vi "DHE_SetControllerParams.vi"(9 "framesperbuffer":i32, 10 "ControllerStatus":T1={"Response"="", "power"=FALSE, "shutter"=FALSE, "artifdata"=FALSE, "idlemode"=FALSE, "reset"=FALSE, "gain"=0, "speed"=0, "resetPCI"=FALSE, "autoshutter"=FALSE, "TempSetPoint"=-110, "multipleextensions"=FALSE, "displayImage"=TRUE, "coadding"=FALSE, "images being coadded"=1, "Operation Mode"=enum."normal", "frames to write"={"subs"=FALSE, "reset"=FALSE, "exposed"=FALSE}, "fawler samples"=1, "write auto"=FALSE, "datatype"="", "frames to display"={"subs"=FALSE, "reset"=FALSE, "exposed"=FALSE}, "sur"=1, "autoclear"=FALSE}) -> ()   [LabVIEW 2016]
uses:
  Common/public/vis/CMN_ContStatus.ctl
  DBSHAND/private/vis/DatabaseHand_Element_Set(bool).vi
  DBSHAND/private/vis/DatabaseHand_Element_Set(U8).vi
  DBSHAND/private/vis/DatabaseHand_Element_Set(I32).vi
  DBSHAND/private/vis/DatabaseHand_Element_Set(string).vi
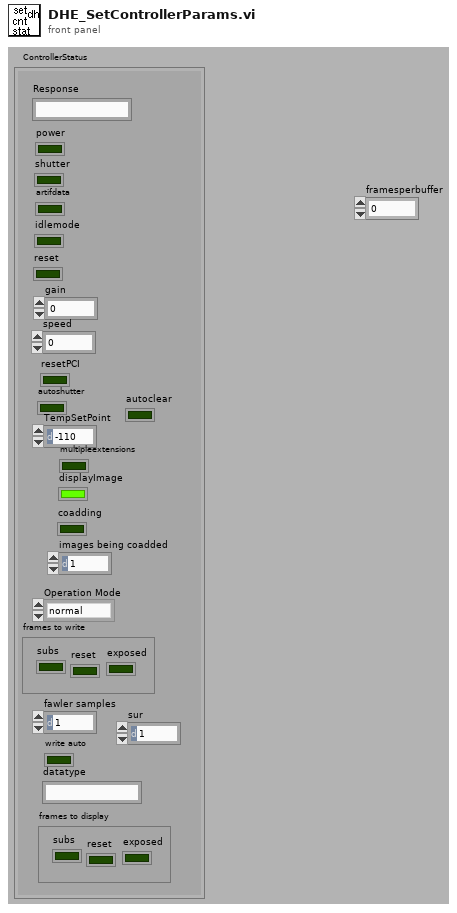
[diagram p1: front panel]
types:
  T1 = typedef "CMN_ContStatus.ctl" = cluster{"Response":string, "power":bool, "shutter":bool, "artifdata":bool, "idlemode":bool, "reset":bool, "gain":u8, "speed":u8, "resetPCI":bool, "autoshutter":bool, "TempSetPoint":i32, "multipleextensions":bool, "displayImage":bool, "coadding":bool, "images being coadded":i32, "Operation Mode":enum16{"normal", "coadd", "fawler"}, "frames to write":cluster{"subs":bool, "reset":bool, "exposed":bool}, "fawler samples":i32, "write auto":bool, "datatype":string, "frames to display":cluster{"subs":bool, "reset":bool, "exposed":bool}, "sur":i32, "autoclear":bool}
  T2 = typedef "DatabaseHand_RefNum.ctl" = refnum<vi>
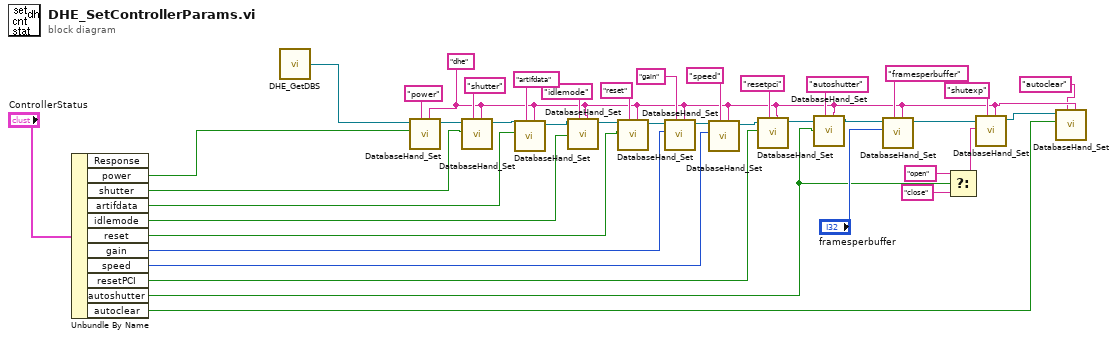
[diagram p0: block diagram]
diagram:
  w2 = "dhe" ("group")
  n1 = Unbundle By Name("ControllerStatus") -> ("power"=w38:bool, "shutter"=w32:bool, "artifdata"=w30:bool, "idlemode"=w28:bool, "reset"=w26:bool, "gain"=w16:u8, "speed"=w15:u8, "resetPCI"=w25:bool, "autoshutter"=w8:bool, "autoclear"=w3:bool)  [unwired: 1 out]
  n2 = call "DHE_GetDBS.vi"() -> ("DHE_DBSRef"=w11:T2)  [unwired: 9 out]
  n3 = call-poly "DatabaseHand_Set.vi"("group"=w2, "name"="power", "value"=w38, "Database RefNum in"=w11) -> ("Database RefNum out"=w37:T2)  [unwired: 4 in, 3 out]
  n4 = call-poly "DatabaseHand_Set.vi"("group"=w2, "name"="shutter", "value"=w32, "Database RefNum in"=w37) -> ("Database RefNum out"=w36:T2)  [unwired: 4 in, 3 out]
  n5 = call-poly "DatabaseHand_Set.vi"("group"=w2, "name"="artifdata", "value"=w30, "Database RefNum in"=w36) -> ("Database RefNum out"=w35:T2)  [unwired: 4 in, 3 out]
  n6 = call-poly "DatabaseHand_Set.vi"("group"=w2, "name"="idlemode", "value"=w28, "Database RefNum in"=w35) -> ("Database RefNum out"=w34:T2)  [unwired: 4 in, 3 out]
  n7 = call-poly "DatabaseHand_Set.vi"("group"=w2, "name"="reset", "value"=w26, "Database RefNum in"=w34) -> ("Database RefNum out"=w21:T2)  [unwired: 4 in, 3 out]
  n8 = call-poly "DatabaseHand_Set.vi"("group"=w2, "name"="gain", "value"=w16, "Database RefNum in"=w21) -> ("Database RefNum out"=w20:T2)  [unwired: 4 in, 3 out]
  n9 = call-poly "DatabaseHand_Set.vi"("group"=w2, "name"="speed", "value"=w15, "Database RefNum in"=w20) -> ("Database RefNum out"=w19:T2)  [unwired: 4 in, 3 out]
  n10 = call-poly "DatabaseHand_Set.vi"("group"=w2, "name"="resetpci", "value"=w25, "Database RefNum in"=w19) -> ("Database RefNum out"=w33:T2)  [unwired: 4 in, 3 out]
  n11 = call-poly "DatabaseHand_Set.vi"("group"=w2, "name"="autoshutter", "value"=w8, "Database RefNum in"=w33) -> ("Database RefNum out"=w14:T2)  [unwired: 4 in, 3 out]
  n12 = call-poly "DatabaseHand_Set.vi"("group"=w2, "name"="framesperbuffer", "value"="framesperbuffer", "Database RefNum in"=w14) -> ("Database RefNum out"=w10:T2)  [unwired: 4 in, 3 out]
  n13 = Select(t="open", s=w8, f="close") -> (s? t:f=w5:string)
  n14 = call-poly "DatabaseHand_Set.vi"("group"=w2, "name"="shutexp", "value"=w5, "Database RefNum in"=w10) -> ("Database RefNum out"=w4:T2)  [unwired: 4 in, 3 out]
  n15 = call-poly "DatabaseHand_Set.vi"("group"=w2, "name"="autoclear", "value"=w3, "Database RefNum in"=w4) -> ()  [unwired: 4 in, 4 out]
